vi "input.vi"(8 "error in":errorcluster, 10 "data table in":T1, 11 "SQLite runtime in":refnum<class "SQLite runtime.lvclass">) -> (0 "error out":errorcluster, 2 "data table out":T1, 3 "SQLite runtime out":refnum<class "SQLite runtime.lvclass">)   [LabVIEW 2014, in "SQLite runtime.lvclass"]
doc: "Provides an interface for reading data from a module at runtime. While this interface performs no operations, a child should provide an override which may read from any open sessions, references, or interfaces."
uses:
  SQLite runtime.lvclass
  <vilib>/NI/Tag Bus/table/data table.ctl
  SQLite runtime.lvclass/SQLite runtime.ctl
  <vilib>/drjdpowell/SQLite Library/SQL Statement/SQL Statement.lvclass/SQL Statement.ctl
  <vilib>/NI/Tag Bus/table/data polymorphs/write one/write Double.vi
  <vilib>/NI/Tag Bus/table/data polymorphs/write one/write Single.vi
  <vilib>/drjdpowell/SQLite Library/SQL Statement/Column DBL.vi
  <vilib>/NI/Tag Bus/table/data polymorphs/write one/write I64.vi
  <vilib>/NI/Tag Bus/table/data polymorphs/write one/write I32.vi
  <vilib>/NI/Tag Bus/table/data polymorphs/write one/write I16.vi
  <vilib>/NI/Tag Bus/table/data polymorphs/write one/write I8.vi
  <vilib>/NI/Tag Bus/table/data polymorphs/write one/write U64.vi
  <vilib>/NI/Tag Bus/table/data polymorphs/write one/write U32.vi
  <vilib>/NI/Tag Bus/table/data polymorphs/write one/write U16.vi
  <vilib>/NI/Tag Bus/table/data polymorphs/write one/write U8.vi
  <vilib>/NI/Tag Bus/table/data polymorphs/write one/write Boolean.vi
  <vilib>/drjdpowell/SQLite Library/SQL Statement/Column I64.vi
  <vilib>/NI/Tag Bus/table/data polymorphs/write one/write String.vi
  <vilib>/drjdpowell/SQLite Library/SQL Statement/Reset (Property).vi
  <vilib>/drjdpowell/SQLite Library/SQL Statement/Column Type.vi
  <vilib>/drjdpowell/SQLite Library/SQL Statement/Reset.vi
  <vilib>/drjdpowell/SQLite Library/SQL Statement/Error Message.vi
  <vilib>/drjdpowell/SQLite Library/SQL Statement/Column String.vi
  <vilib>/drjdpowell/SQLite Library/SQL Statement/SQL Statement.lvclass
  <vilib>/NI/Tag Bus/table/data table.lvlib
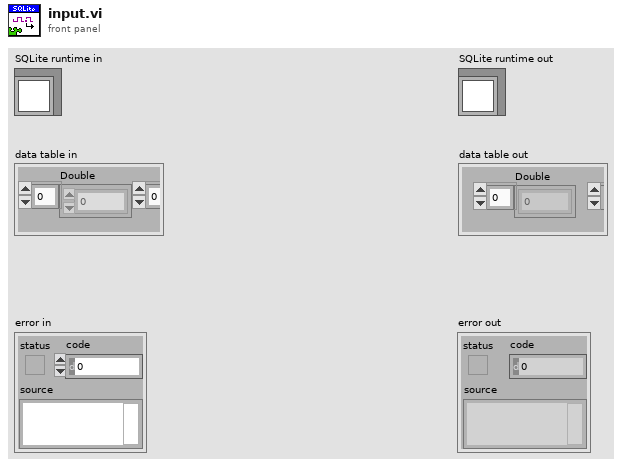
[diagram p1: front panel]
types:
  T1 = typedef "tag bus.lvlib/data table.lvlib/data table.ctl" = cluster{"Double":dbl[], "Single":sgl[], "I64":i64[], "I32":i32[], "I16":i16[], "I8":i8[], "U64":u64[], "U32":u32[], "U16":u16[], "U8":u8[], "Boolean":bool[], "String":string[], "Array of Double":cluster{"DBL Array":dbl[]}[], "Array of Single":cluster{"SGL Array":sgl[]}[], "Array of I64":cluster{"I64 Array":i64[]}[], "Array of I32":cluster{"I32 Array":i32[]}[], "Array of I16":cluster{"I16 Array":i16[]}[], "Array of I8":cluster{"I8 Array":i8[]}[], "Array of U64":cluster{"U64 Array":u64[]}[], "Array of U32":cluster{"U32 Array":u32[]}[], "Array of U16":cluster{"U16 Array":u16[]}[], "Array of U8":cluster{"U8 Array":u8[]}[], "Array of Boolean":cluster{"Boolean Array":bool[]}[], "Array of String":cluster{"String Array":string[]}[]}
  T2 = typedef "tag bus.lvlib/tag descriptor.lvclass/Data Type.ctl" = enum16{"Double", "Single", "I64", "I32", "I16", "I8", "U64", "U32", "U16", "U8", "Boolean", "String", "Array of Double", "Array of Single", "Array of I64", "Array of I32", "Array of I16", "Array of I8", "Array of U64", "Array of U32", "Array of U16", "Array of U8", "Array of Boolean", "Array of String"}
  T3 = typedef "SQLite runtime.lvclass/sqlite type.ctl" = enum16{"DBL", "I64", "String"}
  T4 = cluster{"DCAF Type":T2, "Index":i32, "SQLite Type":T3, "db key":string}[]
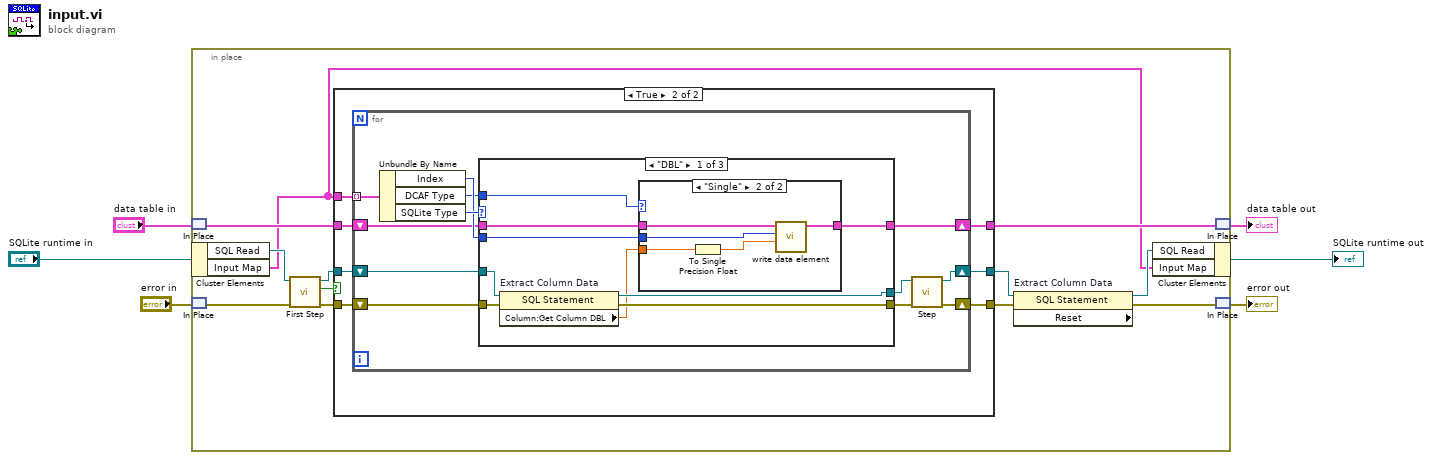
[diagram p0: block diagram]
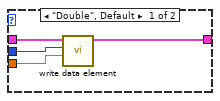
[diagram p3: hidden frame]
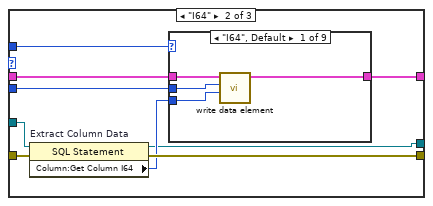
[diagram p4: hidden frame]
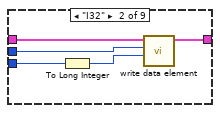
[diagram p5: hidden frame]
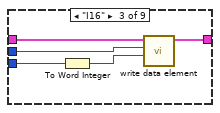
[diagram p6: hidden frame]
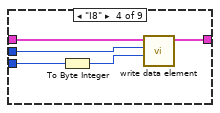
[diagram p7: hidden frame]
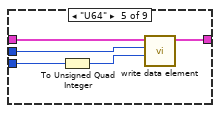
[diagram p8: hidden frame]
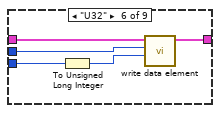
[diagram p9: hidden frame]
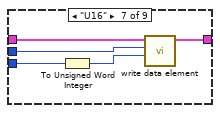
[diagram p10: hidden frame]
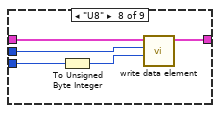
[diagram p11: hidden frame]
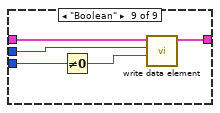
[diagram p12: hidden frame]
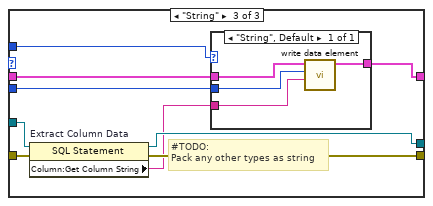
[diagram p13: hidden frame]
diagram:
  n1 = in-place {
    n2 = in-place-match #1("data table in") -> (w9:T1)
    n3 = in-place-cluster #2("SQLite runtime in") -> ("SQL Read"=w18:refnum<class "SQL Statement.lvclass">, "Input Map"=w7:T4)
    n4 = in-place-match #3("error in") -> (w17:errorcluster)
    n5 = call <vilib>:"First Step.vi"("error in (no error)"=w17, "SQL Statement in"=w18) -> ("error out"=w10:errorcluster, "Row returned"=w16:bool, "SQL Statement out"=w15:refnum<class "SQL Statement.lvclass">)  [unwired: 7 in]
    n6 = case shown="True" w16 {
      tunnel: w15 -> [w21 w28]
      tunnel: [w21 w27] -> w14
      tunnel: [w20 w26] -> w11
      tunnel: w10 -> [w20 w25]
      tunnel: w9 -> [w19 w24]
      tunnel: [w19 w23] -> w8
      tunnel: w7 -> [_ w22]
      frame False {
      }
      frame True {
        n7 = for {
          shift-right: [w39] -> w27
          shift-left: w28 -> [w37]
          shift-right: [w40] -> w26
          shift-left: w25 -> [w36]
          shift-right: [w32] -> w23
          shift-left: w24 -> [w33]
          tunnel: w22 -> [w38] mode=indexing
          n8 = Unbundle By Name(w38) -> ("Index"=w34:i32, "DCAF Type"=w31:T2, "SQLite Type"=w35:T3)
          n9 = case shown="\"DBL\"" w35 {
            tunnel: w37 -> [w49 w67 w120]
            tunnel: [w48 w59 w119] -> w29
            tunnel: w36 -> [w47 w66 w118]
            tunnel: [w46 w65 w117] -> w30
            tunnel: w34 -> [w41 w60 w113]
            tunnel: w33 -> [w45 w64 w116]
            tunnel: [w44 w63 w115] -> w32
            tunnel: w31 -> [w42 w61 w112]
            frame "DBL" {
              n10 = property on="Extract Column Data" class="SQL Statement"(reference=w49, error in=w47) -> (reference out=w48:refnum<class "SQL Statement.lvclass">, error out=w46:errorcluster, "Column:Get Column DBL"=w43:dbl)
              n11 = case shown="\"Single\"" w42 {
                tunnel: w45 -> [w53 w58]
                tunnel: [w52 w57] -> w44
                tunnel: w43 -> [w50 w56]
                tunnel: w41 -> [w51 w54]
                frame "Double", Default {
                  n12 = call-poly <vilib>:"write data element.vi"("value"=w50, "index"=w51, "data table in"=w53) -> ("data table out"=w52:T1)  [unwired: 8 in]
                }
                frame "Single" {
                  n13 = To Single Precision Float(number=w56) -> (single precision float=w55:sgl)
                  n14 = call-poly <vilib>:"write data element.vi"("value"=w55, "index"=w54, "data table in"=w58) -> ("data table out"=w57:T1)  [unwired: 8 in]
                }
              }
            }
            frame "I64" {
              n15 = property on="Extract Column Data" class="SQL Statement"(reference=w67, error in=w66) -> (reference out=w59:refnum<class "SQL Statement.lvclass">, error out=w65:errorcluster, "Column:Get Column I64"=w62:i64)
              n16 = case shown="\"I64\", Default" w61 {
                tunnel: w64 -> [w71 w76 w81 w86 w91 w96 w101 w106 w111]
                tunnel: [w70 w75 w80 w85 w90 w95 w100 w105 w110] -> w63
                tunnel: w62 -> [w68 w72 w77 w82 w87 w92 w97 w102 w107]
                tunnel: w60 -> [w69 w74 w79 w84 w89 w94 w99 w104 w109]
                frame "I64", Default {
                  n17 = call-poly <vilib>:"write data element.vi"("value"=w68, "index"=w69, "data table in"=w71) -> ("data table out"=w70:T1)  [unwired: 8 in]
                }
                frame "I32" {
                  n18 = To Long Integer(number=w72) -> (32bit integer=w73:i32)
                  n19 = call-poly <vilib>:"write data element.vi"("value"=w73, "index"=w74, "data table in"=w76) -> ("data table out"=w75:T1)  [unwired: 8 in]
                }
                frame "I16" {
                  n20 = To Word Integer(number=w77) -> (16bit integer=w78:i16)
                  n21 = call-poly <vilib>:"write data element.vi"("value"=w78, "index"=w79, "data table in"=w81) -> ("data table out"=w80:T1)  [unwired: 8 in]
                }
                frame "I8" {
                  n22 = To Byte Integer(number=w82) -> (8bit integer=w83:i8)
                  n23 = call-poly <vilib>:"write data element.vi"("value"=w83, "index"=w84, "data table in"=w86) -> ("data table out"=w85:T1)  [unwired: 8 in]
                }
                frame "U64" {
                  n24 = To Unsigned Quad Integer(1:w87) -> (0:w88:u64)
                  n25 = call-poly <vilib>:"write data element.vi"("value"=w88, "index"=w89, "data table in"=w91) -> ("data table out"=w90:T1)  [unwired: 8 in]
                }
                frame "U32" {
                  n26 = To Unsigned Long Integer(number=w92) -> (unsigned 32bit integer=w93:u32)
                  n27 = call-poly <vilib>:"write data element.vi"("value"=w93, "index"=w94, "data table in"=w96) -> ("data table out"=w95:T1)  [unwired: 8 in]
                }
                frame "U16" {
                  n28 = To Unsigned Word Integer(number=w97) -> (unsigned 16bit integer=w98:u16)
                  n29 = call-poly <vilib>:"write data element.vi"("value"=w98, "index"=w99, "data table in"=w101) -> ("data table out"=w100:T1)  [unwired: 8 in]
                }
                frame "U8" {
                  n30 = To Unsigned Byte Integer(number=w102) -> (unsigned 8bit integer=w103:u8)
                  n31 = call-poly <vilib>:"write data element.vi"("value"=w103, "index"=w104, "data table in"=w106) -> ("data table out"=w105:T1)  [unwired: 8 in]
                }
                frame "Boolean" {
                  n32 = Not Equal To 0?(x=w107) -> (x != 0?=w108:bool)
                  n33 = call-poly <vilib>:"write data element.vi"("value"=w108, "index"=w109, "data table in"=w111) -> ("data table out"=w110:T1)  [unwired: 8 in]
                }
              }
            }
            frame "String" {
              # "#TODO:\nPack any other types as string"
              n34 = property on="Extract Column Data" class="SQL Statement"(reference=w120, error in=w118) -> (reference out=w119:refnum<class "SQL Statement.lvclass">, error out=w117:errorcluster, "Column:Get Column String"=w114:string)
              n35 = case shown="\"String\", Default" w112 {
                tunnel: w116 -> [w124]
                tunnel: [w123] -> w115
                tunnel: w114 -> [w122]
                tunnel: w113 -> [w121]
                frame "String", Default {
                  n36 = call-poly <vilib>:"write data element.vi"("value"=w122, "index"=w121, "data table in"=w124) -> ("data table out"=w123:T1)  [unwired: 8 in]
                }
              }
            }
          }
          n37 = call <vilib>:"Step.vi"("error in (no error)"=w30, "SQL Statement in"=w29) -> ("error out"=w40:errorcluster, "SQL Statement out"=w39:refnum<class "SQL Statement.lvclass">)  [unwired: 7 in, 1 out]
        }
      }
    }
    n38 = property on="Extract Column Data" class="SQL Statement" props=["Reset"](reference=w14, error in=w11) -> (reference out=w13:refnum<class "SQL Statement.lvclass">, error out=w12:errorcluster)  [unwired: 1 out]
    n39 = in-place-cluster #2("SQL Read"=w13, "Input Map"=w7) -> (→"SQLite runtime out":refnum<class "SQLite runtime.lvclass">)
    n40 = in-place-match #1(w8) -> (→"data table out":T1)
    n41 = in-place-match #3(w12) -> (→"error out":errorcluster)
  }
